vi "Dashboard Recieve.vi"(10 "connection ID":refnum<k16>) -> ()   [LabVIEW 2016]
uses:
  Common Code/Dashboard Control Data.ctl
  Common Code/Intake Presets.ctl
  Common Code/Drivetrain Presets.ctl
  Robot Global Data.vi
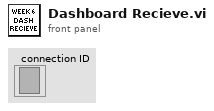
[diagram p1: front panel]
types:
  T1 = typedef "Dashboard Control Data.ctl" = cluster{"Intake Presets":T2, "Drivetrain Presets":T3}
  T2 = typedef "Intake Presets.ctl" = cluster{"Intake Power":dbl, "Outtake Power":dbl}
  T3 = typedef "Drivetrain Presets.ctl" = cluster{"Steer PID output":cluster{"output high":dbl, "output low":dbl}, " Steer PID gains":cluster{"proportional gain (Kc)":dbl, "integral time (Ti, min)":dbl, "derivative time (Td, min)":dbl}, "Gyro Tolerance":dbl}
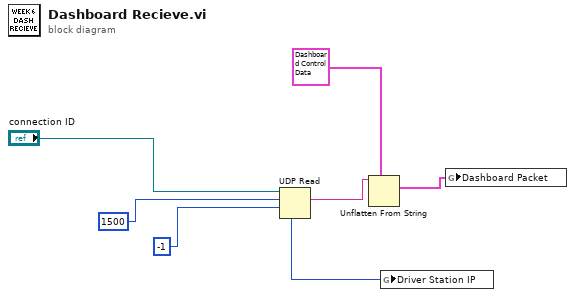
[diagram p0: block diagram]
diagram:
  n1 = UDP Read(connection ID="connection ID", max size (548)=1500, timeout ms (25000)=-1) -> (data out=w3:string, 6:w7:u32)  [unwired: 1 in, 3 out]
  n2 = Unflatten From String(type=T1 {"Intake Presets"={"Intake Power"=0.0, "Outtake Power"=0.0}, "Drivetrain Presets"={"Steer PID output"={"output high"=0.0, "output low"=0.0}, " Steer PID gains"={"proportional gain (Kc)"=0.0, "integral time (Ti, min)"=0.0, "derivative time (Td, min)"=0.0}, "Gyro Tolerance"=0.0}} ("Dashboard Packet"), binary string=w3) -> (value=w1:T1)  [unwired: 3 in, 2 out]
  n3 = global write "Robot Global Data.vi" "Driver Station IP"(w7) -> ()
  n4 = global write "Robot Global Data.vi" "Dashboard Packet"(w1) -> ()
